vi "TDT-Adjust Event List.vi"(9 "Events in":dbl[][](array[numeric]), 11 "Last In":dbl) -> (1 "Events out":dbl[][](array[numeric]), 3 "Last out":dbl)   [LabVIEW 2020]
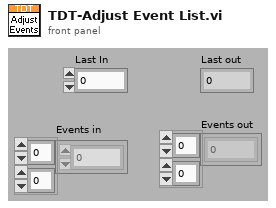
[diagram p1: front panel]
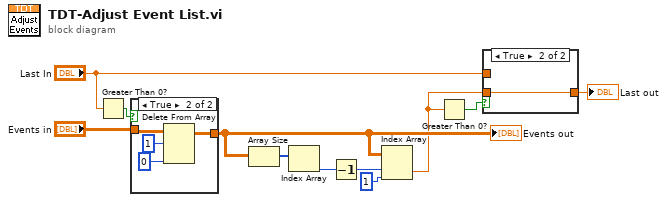
[diagram p0: block diagram]
diagram:
  n1 = Greater Than 0?(x="Last In") -> (x > 0?=w11:bool)
  n2 = case shown="True" w11 {
    tunnel: "Events in" -> [w12 w16]
    tunnel: [w12 w13] -> w9
    frame False {
    }
    frame True {
      n3 = Delete From Array(array=w16, length=1, index (row)=0) -> (array with subset deleted=w13:dbl[][])  [unwired: 1 in, 1 out]
    }
  }
  "Events out" <- w9
  n4 = Array Size(array=w9) -> (size(s)=w8:i32[])
  n5 = Index Array(array=w8) -> (element=w7:i32)  [unwired: 1 in]
  n6 = Decrement(x=w7) -> (x-1=w6:i32)
  n7 = Index Array(array=w9, index (row)=w6, index (col)=1 ("disabled index (col)")) -> (element=w4:dbl)
  n8 = Greater Than 0?(x=w4) -> (x > 0?=w5:bool)
  n9 = case shown="True" w5 {
    tunnel: w4 -> [_ w18]
    tunnel: [w17 w18] -> w2
    tunnel: "Last In" -> [w17 _]
    frame False {
    }
    frame True {
    }
  }
  "Last out" <- w2
